vi "test_MonoMoveAndGetMirrorPosition.vi"(0 "device selection":enum16{"monochromator", "CCD", "SCD"}(ring), 1 "Test should pass":bool=TRUE, 5 "set-up a connection":bool=TRUE, 9 "tear down connection":bool=TRUE, 11 "error in":errorcluster, 12 "Delay between send and receive [ms]":i32=100) -> (4 "first loop":i32, 6 "first loop 2":i32, 8 "first loop 3":i32, 10 "log-file path":path, 15 "error out":errorcluster)   [LabVIEW 2023, in "horiba.test.lvlib"]
uses:
  Classes/Mono/Monochromator.lvclass
  <vilib>/addons/_JKI Toolkits/Caraya/classes/Assert/Assert Equal Value and Type_Variant.vi
  <vilib>/addons/_JKI Toolkits/Caraya/classes/Assert/Assert True.vi
  <vilib>/addons/_JKI Toolkits/Caraya/classes/Assert/Assert Not Error.vi
  horiba.test.lvlib
  <vilib>/addons/_JKI Toolkits/Caraya/classes/Test/Test.lvclass
  <vilib>/addons/_JKI Toolkits/Caraya/classes/Assert/Assert.lvclass
  Classes/horiba.lvlib
  <vilib>/Hampel Software Engineering/HSE Logger/hse-logger.lvlib
  C:/Projects/Horiba/horiba-labview-sdk/Source/Classes/GenericDevice/GenericDevice.lvclass
  C:/Projects/Horiba/horiba-labview-sdk/Source/Classes/Mono/Monochromator.lvclass
panel:
  # "Connector Pane"
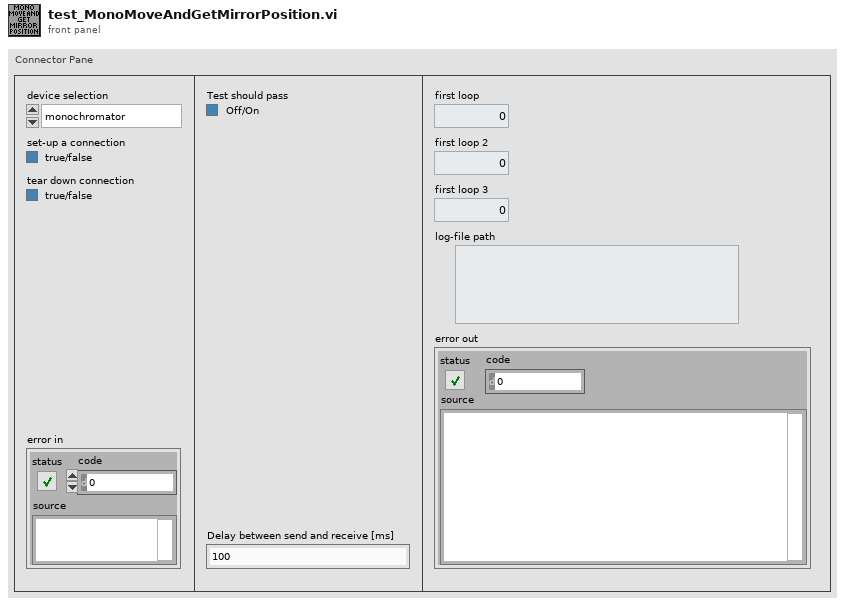
[diagram p1: front panel]
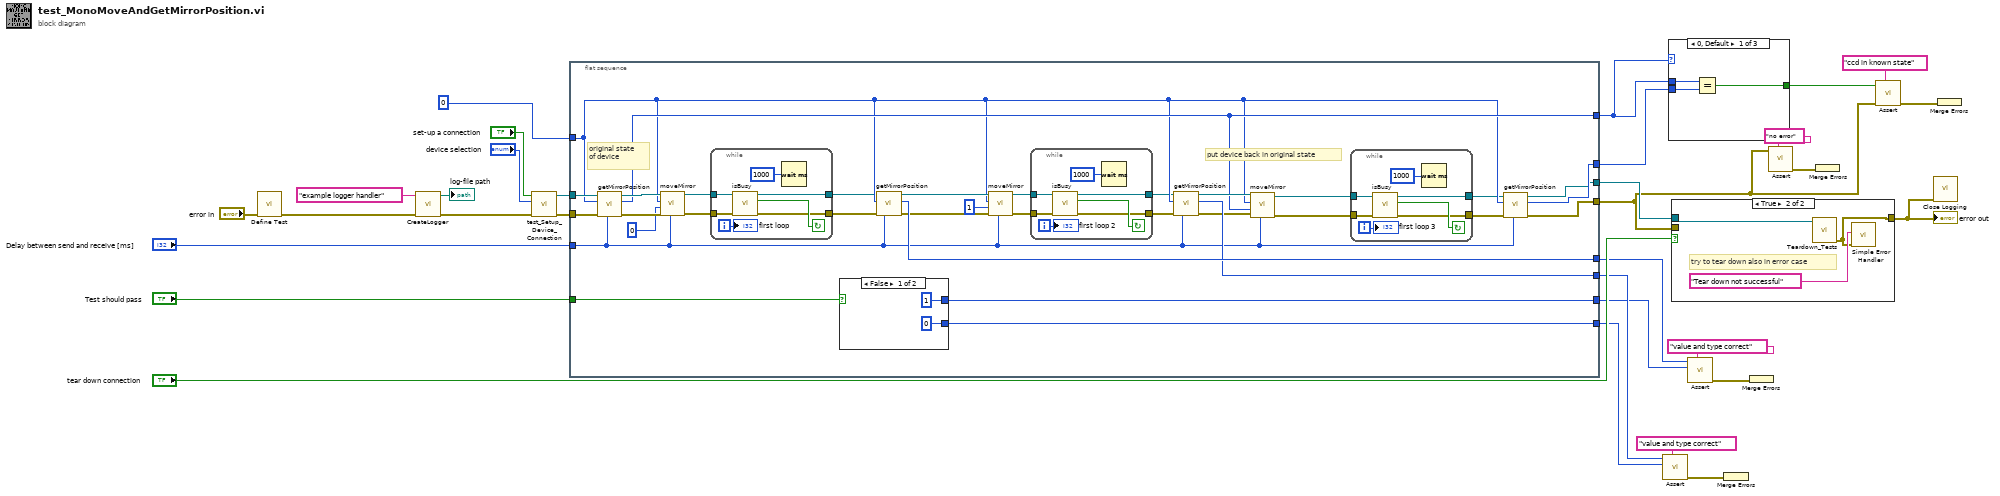
[diagram p0: block diagram]
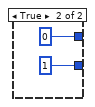
[diagram p2: hidden frame]
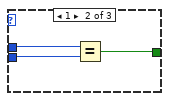
[diagram p3: hidden frame]
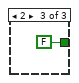
[diagram p4: hidden frame]
diagram:
  n1 = call <vilib>:"Define Test.vi"("error in (no error)"="error in") -> ("error out"=w10:errorcluster)  [unwired: 9 in, 1 out]
  n2 = call "CreateLogger.vi"("error in (no error)"=w10, "Handler Name"="example logger handler") -> ("error out"=w9:errorcluster, "log-file path"=→"log-file path":path)  [unwired: 8 in]
  n3 = call "test_Setup_Device_Connection.vi"("error in (no error)"=w9, "device selection"="device selection", "set-up a connection"="set-up a connection") -> ("error out"=w15:errorcluster, "Monochromator out"=w13:refnum<class "Monochromator.lvclass">)  [unwired: 5 in, 2 out]
  n4 = flat-sequence {
    tunnel: w15 -> [w60]
    tunnel: w13 -> [w61]
    tunnel: [w49] -> w6
    tunnel: "Test should pass" -> [w64]
    tunnel: [w50] -> w22
    tunnel: [w54] -> w21
    tunnel: [w63] -> w20
    tunnel: [w57] -> w19
    tunnel: [w62] -> w18
    tunnel: [w48] -> w5
    tunnel: [w51] -> w4
    tunnel: "Delay between send and receive [ms]" -> [w46]
    tunnel: 0 -> [w47]
    frame #0 {
      # "put device back in original state"
      # "original state of device"
      n5 = call "getMirrorPosition.vi"("Delay between send and receive [ms]"=w46, "error in (no error)"=w60, "locationId"=w47, "Monochromator in"=w61) -> ("error out"=w58:errorcluster, "position"=w48:i32, "Monochromator out"=w59:refnum<class "Monochromator.lvclass">)  [unwired: 5 in]
      n6 = call "moveMirror.vi"("Delay between send and receive [ms]"=w46, "error in (no error)"=w58, "position"=0, "locationId"=w47, "Monochromator in"=w59) -> ("error out"=w43:errorcluster, "Monochromator out"=w45:refnum<class "Monochromator.lvclass">)  [unwired: 3 in, 2 out]
      n7 = while {
        tunnel: w45 -> [w76]
        tunnel: [w75] -> w44
        tunnel: w43 -> [w74]
        tunnel: [w73] -> w42
        i -> [w72]
        stop <- w78 continue-if-true
        n8 = call "isBusy.vi"("error in (no error)"=w74, "Monochromator in"=w76) -> ("error out"=w73:errorcluster, "mono is busy?"=w78:bool, "Monochromator out"=w75:refnum<class "Monochromator.lvclass">)  [unwired: 7 in]
        n9 = Wait (ms)(milliseconds to wait=u32 1000) -> ()  [unwired: 1 out]
        "first loop" <- w72
      }
      n10 = case shown="False" w64 {
        tunnel: [0 1] -> w63
        tunnel: [1 0] -> w62
        frame False {
        }
        frame True {
        }
      }
      n11 = call "getMirrorPosition.vi"("Delay between send and receive [ms]"=w46, "error in (no error)"=w42, "locationId"=w47, "Monochromator in"=w44) -> ("error out"=w55:errorcluster, "position"=w57:i32, "Monochromator out"=w56:refnum<class "Monochromator.lvclass">)  [unwired: 5 in]
      n12 = call "moveMirror.vi"("Delay between send and receive [ms]"=w46, "error in (no error)"=w55, "position"=1, "locationId"=w47, "Monochromator in"=w56) -> ("error out"=w39:errorcluster, "Monochromator out"=w41:refnum<class "Monochromator.lvclass">)  [unwired: 3 in, 2 out]
      n13 = while {
        tunnel: w41 -> [w87]
        tunnel: [w86] -> w40
        tunnel: w39 -> [w85]
        tunnel: [w84] -> w38
        i -> [w83]
        stop <- w89 continue-if-true
        n14 = call "isBusy.vi"("error in (no error)"=w85, "Monochromator in"=w87) -> ("error out"=w84:errorcluster, "mono is busy?"=w89:bool, "Monochromator out"=w86:refnum<class "Monochromator.lvclass">)  [unwired: 7 in]
        n15 = Wait (ms)(milliseconds to wait=u32 1000) -> ()  [unwired: 1 out]
        "first loop 2" <- w83
      }
      n16 = call "getMirrorPosition.vi"("Delay between send and receive [ms]"=w46, "error in (no error)"=w38, "locationId"=w47, "Monochromator in"=w40) -> ("error out"=w52:errorcluster, "position"=w54:i32, "Monochromator out"=w53:refnum<class "Monochromator.lvclass">)  [unwired: 5 in]
      n17 = call "moveMirror.vi"("Delay between send and receive [ms]"=w46, "error in (no error)"=w52, "position"=w48, "locationId"=w47, "Monochromator in"=w53) -> ("error out"=w35:errorcluster, "Monochromator out"=w37:refnum<class "Monochromator.lvclass">)  [unwired: 3 in, 2 out]
      n18 = while {
        tunnel: w37 -> [w69]
        tunnel: [w68] -> w36
        tunnel: w35 -> [w67]
        tunnel: [w66] -> w34
        i -> [w65]
        stop <- w71 continue-if-true
        n19 = call "isBusy.vi"("error in (no error)"=w67, "Monochromator in"=w69) -> ("error out"=w66:errorcluster, "mono is busy?"=w71:bool, "Monochromator out"=w68:refnum<class "Monochromator.lvclass">)  [unwired: 7 in]
        n20 = Wait (ms)(milliseconds to wait=u32 1000) -> ()  [unwired: 1 out]
        "first loop 3" <- w65
      }
      n21 = call "getMirrorPosition.vi"("Delay between send and receive [ms]"=w46, "error in (no error)"=w34, "locationId"=w47, "Monochromator in"=w36) -> ("error out"=w49:errorcluster, "position"=w51:i32, "Monochromator out"=w50:refnum<class "Monochromator.lvclass">)  [unwired: 5 in]
    }
  }
  n22 = call-poly <vilib>:"Assert.vi"("Label"="value and type correct" ("Label (VI Title)"), "Y"=w20, "X"=w21) -> ("error out"=w30:errorcluster)  [unwired: 7 in, 1 out]
  n23 = case shown="0, Default" w5 {
    tunnel: w5 -> [w92 w95 _]
    tunnel: w4 -> [w91 w94 _]
    tunnel: [w90 w93 FALSE] -> w3
    frame 0, Default {
      n24 = Equal?(x=w92, y=w91) -> (x = y?=w90:bool)
    }
    frame 1 {
      n25 = Equal?(x=w95, y=w94) -> (x = y?=w93:bool)
    }
    frame 2 {
    }
  }
  n26 = case shown="True" "tear down connection" {
    tunnel: w22 -> [_ w99]
    tunnel: [w97 w98] -> w2
    tunnel: w6 -> [w97 _]
    frame False {
    }
    frame True {
      # "try to tear down also in error case"
      n27 = call "Teardown_Tests.vi"("horiba.lvlib:GenericDevice"=w99) -> ("error out"=w98:errorcluster)  [unwired: 9 in, 1 out]
      n28 = call <vilib>:"Simple Error Handler.vi"("error source (\" \")"="Tear down not successful" ("error source (\" \")"), "error in (no error)"=w98) -> ()  [unwired: 3 in, 5 out]
    }
  }
  "error out" <- w2
  n29 = call-poly <vilib>:"Assert.vi"("Label"="value and type correct" ("Label (VI Title)"), "Y"=w18, "X"=w19) -> ("error out"=w29:errorcluster)  [unwired: 7 in, 1 out]
  n30 = Merge Errors(w30) -> ()  [unwired: 1 out]
  n31 = Merge Errors(w29) -> ()  [unwired: 1 out]
  n32 = call-poly <vilib>:"Assert.vi"("Label"="no error" ("Label (VI Title)"), "Not Error?"=w6) -> ("error out"=w24:errorcluster)  [unwired: 8 in, 1 out]
  n33 = Merge Errors(w24) -> ()  [unwired: 1 out]
  n34 = call-poly <vilib>:"Assert.vi"("Label"="ccd in known state" ("Label (VI Title)"), "error in (no error)"=w6, "True?"=w3) -> ("error out"=w8:errorcluster)  [unwired: 7 in, 1 out]
  n35 = call <vilib>:"Close Logging.vi"("error in"=w2) -> ()  [unwired: 10 in, 1 out]
  n36 = Merge Errors(w8) -> ()  [unwired: 1 out]
